vi "Cannon Finish.vi"   [LabVIEW 2013]
types:
  T1 = typedef "WPI_AnalogChannelDevRef.ctl" = cluster{"DevStatus":errorcluster, "Analog Module":T2, "Analog Channel":T3}
  T2 = typedef "FPGA_TypedefAnalogModule.ctl" = enum16{"Analog Module 1", "Analog Module 2"}
  T3 = typedef "FPGA_AIChannel.ctl" = enum8{"AI 1", "AI 2", "AI 3", "AI 4", "AI 5", "AI 6", "AI 7", "AI 8", "Invalid"}
  T4 = typedef "WPI_SolenoidDevRef.ctl" = cluster{"DevStatus":errorcluster, "Solenoid Module":T5, "Forward Solenoid Channel":T6, "Reverse Solenoid Channel":T6}
  T5 = typedef "FPGA_TypedefSolenoidModule.ctl" = enum16{"Solenoid Module 1", "Solenoid Module 2"}
  T6 = typedef "WPI_SolenoidChannel.ctl" = enum8{"Solenoid 1", "Solenoid 2", "Solenoid 3", "Solenoid 4", "Solenoid 5", "Solenoid 6", "Solenoid 7", "Solenoid 8", "Invalid"}
  T7 = typedef "WPI_ServoDeviceRef.ctl" = cluster{"DeviceStatus":errorcluster, "Digital Module":T8, "PWM Channel":T9, "DeadBand":T10}
  T8 = typedef "FPGA_TypedefDigitalModule.ctl" = enum16{"Digital Module 1", "Digital Module 2"}
  T9 = typedef "FPGA_DIOPWMChannel.ctl" = enum8{"PWM 1", "PWM 2", "PWM 3", "PWM 4", "PWM 5", "PWM 6", "PWM 7", "PWM 8", "PWM 9", "PWM 10", "Invalid"}
  T10 = typedef "WPI_PWMDeadband.ctl" = cluster{"Name":string, "maxPositivePwm":i32, "minPositivePwm":i32, "centerPwm":i32, "maxNegativePwm":i32, "minNegativePwm":i32, "angularRange":u16}
  T11 = typedef "WPI_DigitalInputDevRef.ctl" = cluster{"DevStatus":errorcluster, "DIO Channel":T12, "Digital Module":T8}
  T12 = typedef "FPGA_DIOChannel.ctl" = enum8{"DIO 1", "DIO 2", "DIO 3", "DIO 4", "DIO 5", "DIO 6", "DIO 7", "DIO 8", "DIO 9", "DIO 10", "DIO 11", "DIO 12", "DIO 13", "DIO 14", "Invalid"}
  T13 = typedef "WPI_GyroDevRef.ctl" = cluster{"DevStatus":errorcluster, "Analog Module":T2, "Analog Channel":T3, "Offset":dbl, "Gain (VoltsPerDegree/Second)":dbl}
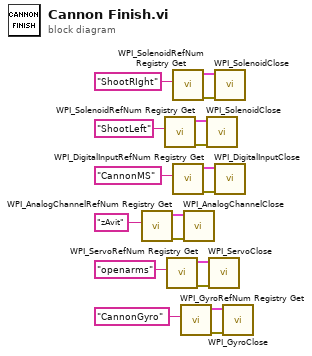
[diagram p0: block diagram]
diagram:
  n1 = call <vilib>:"WPI_AnalogChannelRefNum Registry Get.vi"("refnum name"="zAvit") -> ("error out"=w7:errorcluster, "AIDeviceRef"=w6:T1)  [unwired: 9 in]
  n2 = call <vilib>:"WPI_SolenoidRefNum Registry Get.vi"("refnum name"="ShootLeft") -> ("error out"=w11:errorcluster, "SolenoidDevRef"=w10:T4)  [unwired: 9 in]
  n3 = call <vilib>:"WPI_ServoRefNum Registry Get.vi"("refnum name"="openarms") -> ("error out"=w5:errorcluster, "ServoDeviceRef"=w4:T7)  [unwired: 9 in]
  n4 = call <vilib>:"WPI_SolenoidRefNum Registry Get.vi"("refnum name"="ShootRIght") -> ("error out"=w13:errorcluster, "SolenoidDevRef"=w12:T4)  [unwired: 9 in]
  n5 = call <vilib>:"WPI_DigitalInputRefNum Registry Get.vi"("refnum name"="CannonMS") -> ("error out"=w9:errorcluster, "DigitalInputDevRef"=w8:T11)  [unwired: 9 in]
  n6 = call "WPI_GyroRefNum Registry Get.vi"("refnum name"="CannonGyro") -> ("error out"=w2:errorcluster, "GyroDevRef"=w3:T13)  [unwired: 9 in]
  n7 = call <vilib>:"WPI_AnalogChannelClose.vi"("error in (no error)"=w7, "AIDeviceRef"=w6) -> ()  [unwired: 9 in, 1 out]
  n8 = call <vilib>:"WPI_SolenoidClose.vi"("error in (no error)"=w11, "SolenoidDevRef"=w10) -> ()  [unwired: 9 in, 1 out]
  n9 = call <vilib>:"WPI_ServoClose.vi"("error in (no error)"=w5, "MotorControlDevRef"=w4) -> ()  [unwired: 9 in, 1 out]
  n10 = call <vilib>:"WPI_SolenoidClose.vi"("error in (no error)"=w13, "SolenoidDevRef"=w12) -> ()  [unwired: 9 in, 1 out]
  n11 = call <vilib>:"WPI_DigitalInputClose.vi"("error in (no error)"=w9, "DigitalInputDevRef"=w8) -> ()  [unwired: 9 in, 1 out]
  n12 = call "WPI_GyroClose.vi"("error in (no error)"=w2, "GyroDevRef"=w3) -> ()  [unwired: 9 in, 1 out]
